vi "Receive Vision Packet.vi"(8 "error IO":errorcluster, 10 "Packet":string) -> ()   [LabVIEW 2013]
uses:
  Common Code/Vision Packet.ctl
  Common Code/Goal Info.ctl
  Robot Global Data.vi
  <vilib>/Rock Robotics/WPI/Gyro/WPI_GyroRefNum Registry Get.vi
  <vilib>/Rock Robotics/WPI/Gyro/WPI_GyroGetAngle.vi
panel:
  out "Current Time":u32(graph)
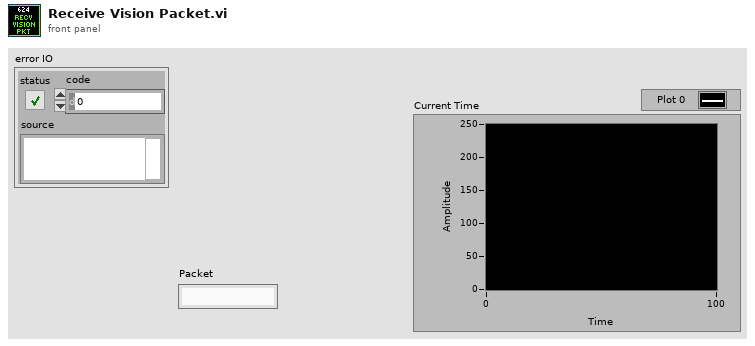
[diagram p1: front panel]
types:
  T1 = typedef "Vision Packet.ctl" = cluster{"Gyro":dbl, "Vision Target":T2, "Timestamp":u32, "Left Goal":T2, "Right Goal":T2}
  T2 = typedef "Goal Info.ctl" = cluster{"Found?":bool, "Target Center":cluster{"X":dbl, "Y":dbl}, "Distance (ft)":dbl, "Hot?":bool, "Left?":bool, "Camera":i16}
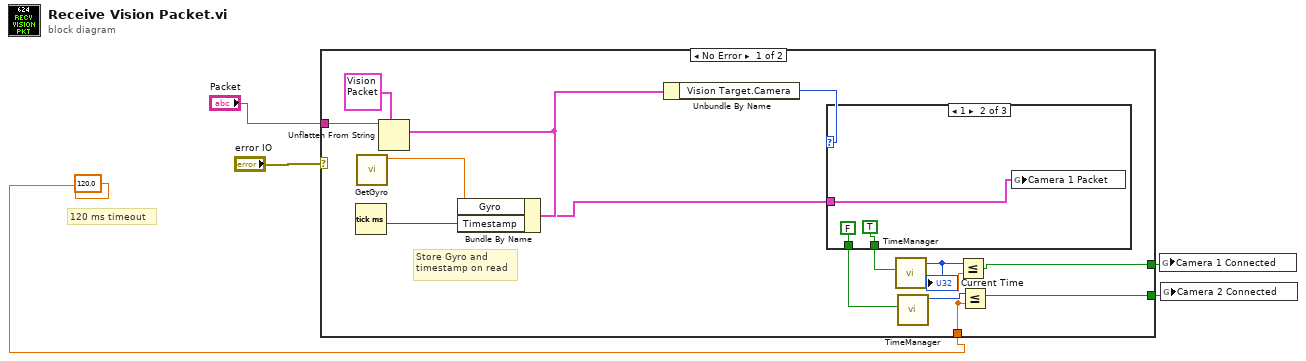
[diagram p0: block diagram]
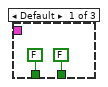
[diagram p2: hidden frame]
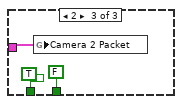
[diagram p3: hidden frame]
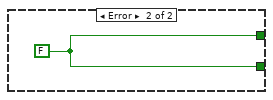
[diagram p4: hidden frame]
diagram:
  # "120 ms timeout"
  n1 = case shown="No Error" "error IO" {
    tunnel: [w8 w28] -> w5
    tunnel: [w7 w28] -> w4
    tunnel: 120.0 ("Numeric") -> [w9 _]
    tunnel: "Packet" -> [w6 _]
    frame No Error {
      # "Store Gyro and\ntimestamp on read"
      n2 = Tick Count (ms)() -> (millisecond timer value=w17:u32)
      n3 = call "GetGyro.vi"() -> ("Angle"=w18:dbl)  [unwired: 9 in, 2 out]
      n4 = Unflatten From String(type=T1 {"Gyro"=0.0, "Vision Target"={"Found?"=FALSE, "Target Center"={"X"=0.0, "Y"=0.0}, "Distance (ft)"=0.0, "Hot?"=FALSE, "Left?"=FALSE, "Camera"=0}, "Timestamp"=0, "Left Goal"={"Found?"=FALSE, "Target Center"={"X"=0.0, "Y"=0.0}, "Distance (ft)"=0.0, "Hot?"=FALSE, "Left?"=FALSE, "Camera"=0}, "Right Goal"={"Found?"=FALSE, "Target Center"={"X"=0.0, "Y"=0.0}, "Distance (ft)"=0.0, "Hot?"=FALSE, "Left?"=FALSE, "Camera"=0}} ("output cluster"), binary string=w6) -> (value=w16:T1)  [unwired: 3 in, 2 out]
      n5 = Bundle By Name(cluster=w16, "Gyro"=w18, "Timestamp"=w17) -> (w14:T1)
      n6 = Unbundle By Name(w16) -> ("Vision Target.Camera"=w15:i16)
      n7 = case shown="1" w15 {
        tunnel: w14 -> [_ w22 w25]
        tunnel: [FALSE TRUE FALSE] -> w13
        tunnel: [FALSE FALSE TRUE] -> w12
        frame Default {
        }
        frame 1 {
          n8 = global write "Robot Global Data.vi" "Camera 1 Packet"(w22) -> ()
        }
        frame 2 {
          n9 = global write "Robot Global Data.vi" "Camera 2 Packet"(w25) -> ()
        }
      }
      n10 = call "TimeManager.vi"("Reset?"=w13) -> ("Time Since Reset"=w11:u32)  [unwired: 9 in, 1 out]
      "Current Time" <- w11
      n11 = call "TimeManager.vi"("Reset?"=w12) -> ("Time Since Reset"=w10:u32)  [unwired: 9 in, 1 out]
      n12 = Less Or Equal?(x=w11, y=w9) -> (x <= y?=w8:bool)
      n13 = Less Or Equal?(x=w10, y=w9) -> (x <= y?=w7:bool)
    }
    frame Error {
      w28 = FALSE
    }
  }
  n14 = global write "Robot Global Data.vi" "Camera 1 Connected"(w5) -> ()
  n15 = global write "Robot Global Data.vi" "Camera 2 Connected"(w4) -> ()
